vi "prepDataForDisplay.vi"(8 "samplingRate":dbl, 9 "dataToRead":u32, 10 "Array in":i16[][](array[numeric]), 11 "Display 1":cluster{"ChArray":bool[]}) -> (3 "Array out 3":i16[][](array[numeric]))   [LabVIEW 2017]
panel:
  out "Array":i32[](array[numeric])
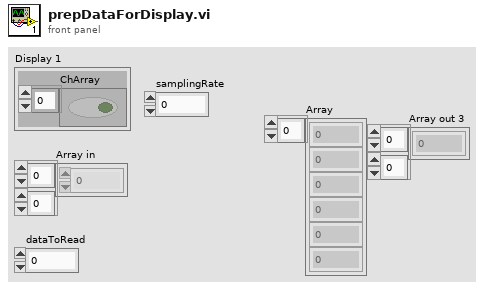
[diagram p1: front panel]
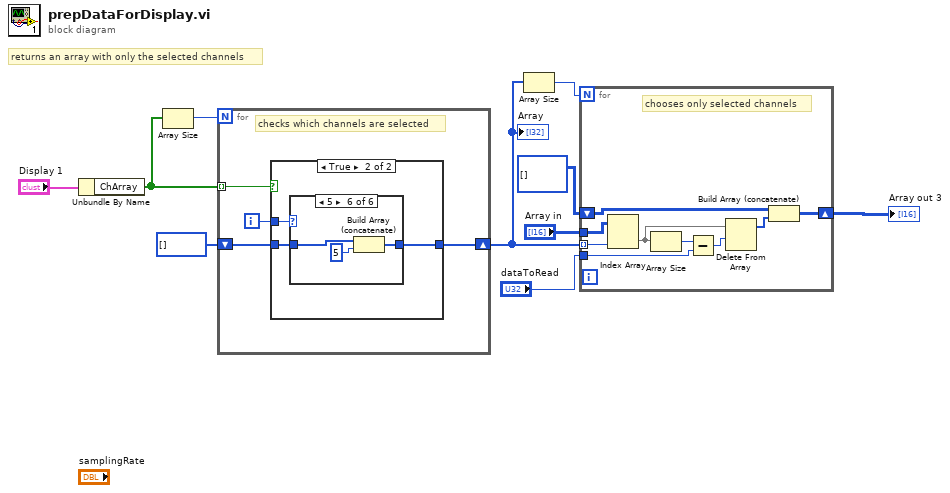
[diagram p0: block diagram]
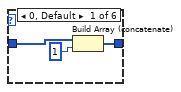
[diagram p3: hidden frame]
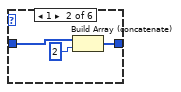
[diagram p4: hidden frame]
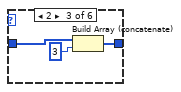
[diagram p5: hidden frame]
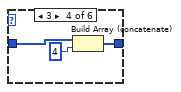
[diagram p6: hidden frame]
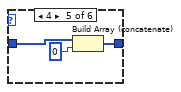
[diagram p7: hidden frame]
diagram:
  # "returns an array with only the selected channels"
  n1 = Unbundle By Name("Display 1") -> ("ChArray"=w8:bool[])
  n2 = Array Size(array=w8) -> (size(s)=w9:i32)
  n3 = for {
    N: w9 -> [_]
    tunnel: w8 -> [w12] mode=indexing
    shift-right: [w13] -> w5
    shift-left: i32[] [] -> [w14]
    i -> [w11]
    # "checks which channels are selected"
    n4 = case shown="True" w12 {
      tunnel: w14 -> [w15 w18]
      tunnel: [w15 w17] -> w13
      tunnel: w11 -> [_ w16]
      frame False {
      }
      frame True {
        n5 = case shown="5" w16 {
          tunnel: w18 -> [w21 w24 w27 w30 w33 w36]
          tunnel: [w20 w23 w26 w29 w32 w35] -> w17
          frame 0, Default {
            n6 = Build Array (concatenate)(w21, 1) -> (w20:i32[])
          }
          frame 1 {
            n7 = Build Array (concatenate)(w24, 2) -> (w23:i32[])
          }
          frame 2 {
            n8 = Build Array (concatenate)(w27, 3) -> (w26:i32[])
          }
          frame 3 {
            n9 = Build Array (concatenate)(w30, 4) -> (w29:i32[])
          }
          frame 4 {
            n10 = Build Array (concatenate)(w33, 0) -> (w32:i32[])
          }
          frame 5 {
            n11 = Build Array (concatenate)(w36, 5) -> (w35:i32[])
          }
        }
      }
    }
  }
  "Array" <- w5
  n12 = Array Size(array=w5) -> (size(s)=w6:i32)
  n13 = for {
    N: w6 -> [_]
    tunnel: w5 -> [w41] mode=indexing
    tunnel: "Array in" -> [w42]
    tunnel: "dataToRead" -> [w40]
    shift-right: [w38] -> w2
    shift-left: i16[][] [] -> [w37]
    # "chooses only selected channels"
    n14 = Index Array(array=w42, index (col)=w41) -> (element=w43:i16[])  [unwired: 1 in]
    n15 = Array Size(array=w43) -> (size(s)=w44:i32)
    n16 = Subtract(x=w44, y=w40) -> (x-y=w45:u32)
    n17 = Delete From Array(array=w43, length=w45) -> (array with subset deleted=w39:i16[])  [unwired: 1 in, 1 out]
    n18 = Build Array (concatenate)(w37, w39) -> (w38:i16[][])
  }
  "Array out 3" <- w2
